vi "Get Monitor from Rectangle.vi"(8 "error in (no error)":errorcluster, 11 "monitor rect":T1) -> (0 "error out":errorcluster, 3 "HMon":u32)   [LabVIEW 2026, in "MacroAssert.lvlib" / "Win Util.lvlib"]
doc: "This VI will find the coordinates of the upper left and lower right corners of the window identified by the 'window refnum' parameter. Coordinate values are in pixels, relative to the upper left corner of the screen. The 'window refnum' can be obtained by using 'Get Window RefNum.vi'."
uses:
  Win Util.lvlib
  user32.dll
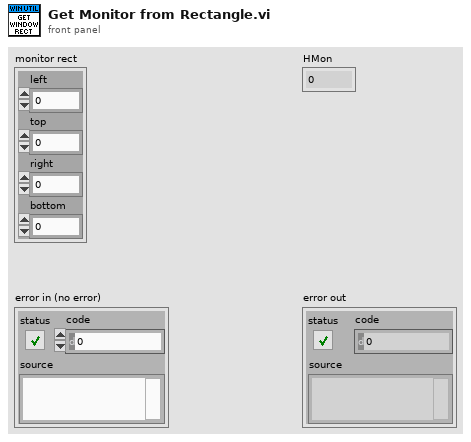
[diagram p1: front panel]
types:
  T1 = cluster{"left":i16, "top":i16, "right":i16, "bottom":i16}
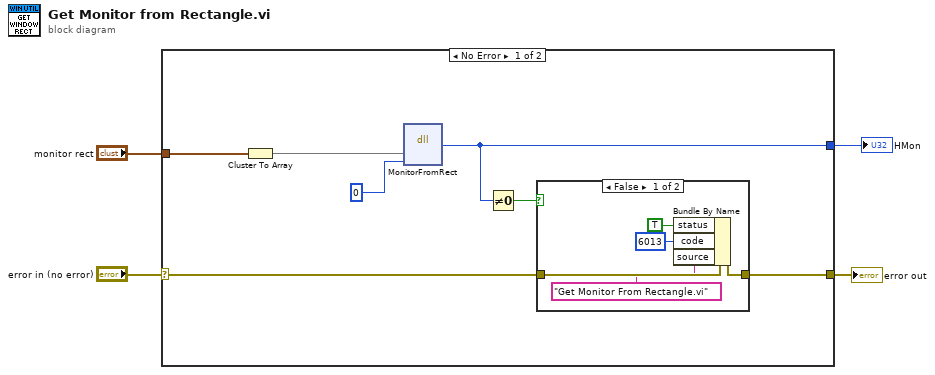
[diagram p0: block diagram]
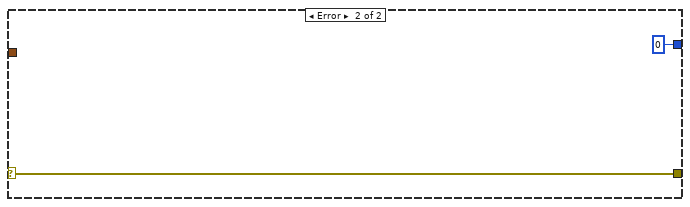
[diagram p3: hidden frame]
diagram:
  n1 = case shown="No Error" "error in (no error)" {
    selector: "error in (no error)" -> [w11 w19]
    tunnel: [w5 u32 0 ("Return Value")] -> w1
    tunnel: [w10 w19] -> w4
    tunnel: "monitor rect" -> [w9 _]
    frame No Error {
      n2 = Cluster To Array(cluster=w9) -> (array=w7:i16[])
      n3 = dll-call lib="user32.dll" fn="MonitorFromRect"("RECT"=w7, "dwFlags"=u32 0) -> ("Return Value"=w5:u32)  [unwired: 3 in, 4 out]
      n4 = Not Equal To 0?(x=w5) -> (x != 0?=w6:bool)
      n5 = case shown="False" w6 {
        tunnel: w11 -> [w16 w17]
        tunnel: [w15 w17] -> w10
        frame False {
          n6 = Bundle By Name(cluster=w16, "status"=TRUE ("show call chain? (False)"), "code"=6013, "source"="Get Monitor From Rectangle.vi") -> (w15:errorcluster)
        }
        frame True {
        }
      }
    }
    frame Error {
    }
  }
  "error out" <- w4
  "HMon" <- w1
